vi "animated ranked results.vi"(0 "cases CSV":string[][](array[string]), 5 "US data":T1, 7 "Populations":i32[](array[numeric]), 9 "deaths CSV":string[][](array[string]), 11 "Countries":string[](array[string])) -> ()   [LabVIEW 2019]
panel:
  in  "Select Country":u16(ring) items=["Afghanistan", "Albania", "Algeria", "Andorra", "Angola", "Antigua and Barbuda", "Argentina", "Armenia", "Australia, Australian Capital Territory", "Australia, New South Wales", "Australia, Northern Territory", "Australia, Queensland", "Australia, South Australia", "Australia, Tasmania", "Australia, Victoria", "Australia, Western Australia", "Austria", "Azerbaijan", "Bahamas", "Bahrain", "Bangladesh", "Barbados", "Belarus", "Belgium", "Benin", "Bhutan", "Bolivia", "Bosnia and Herzegovina", "Brazil", "Brunei", "Bulgaria", "Burkina Faso", "Cabo Verde", "Cambodia", "Cameroon", "Canada, Alberta", "Canada, British Columbia", "Canada, Grand Princess", "Canada, Manitoba", "Canada, New Brunswick", "Canada, Newfoundland and Labrador", "Canada, Nova Scotia", "Canada, Ontario", "Canada, Prince Edward Island", "Canada, Quebec", "Canada, Saskatchewan", "Central African Republic", "Chad", "Chile", "China, Anhui", "China, Beijing", "China, Chongqing", "China, Fujian", "China, Gansu", "China, Guangdong", "China, Guangxi", "China, Guizhou", "China, Hainan", "China, Hebei", "China, Heilongjiang", "China, Henan", "China, Hong Kong", "China, Hubei", "China, Hunan", "China, Inner Mongolia", "China, Jiangsu", "China, Jiangxi", "China, Jilin", "China, Liaoning", "China, Macau", "China, Ningxia", "China, Qinghai", "China, Shaanxi", "China, Shandong", "China, Shanghai", "China, Shanxi", "China, Sichuan", "China, Tianjin", "China, Tibet", "China, Xinjiang", "China, Yunnan", "China, Zhejiang", "Colombia", "Congo (Brazzaville)", "Congo (Kinshasa)", "Costa Rica", "Cote d'Ivoire", "Croatia", "Diamond Princess", "Cuba", "Cyprus", "Czechia", "Denmark, Faroe Islands", "Denmark, Greenland", "Denmark", "Djibouti", "Dominican Republic", "Ecuador", "Egypt", "El Salvador", "Equatorial Guinea", "Eritrea", "Estonia", "Eswatini", "Ethiopia", "Fiji", "Finland", "France, French Guiana", "France, French Polynesia", "France, Guadeloupe", "France, Mayotte", "France, New Caledonia", "France, Reunion", "France, Saint Barthelemy", "France, St Martin", "France, Martinique", "France", "Gabon", "Gambia", "Georgia", "Germany", "Ghana", "Greece", "Guatemala", "Guinea", "Guyana", "Haiti", "Holy See", "Honduras", "Hungary", "Iceland", "India", "Indonesia", "Iran", "Iraq", "Ireland", "Israel", "Italy", "Jamaica", "Japan", "Jordan", "Kazakhstan", "Kenya", "\"Korea", "Kuwait", "Kyrgyzstan", "Latvia", "Lebanon", "Liberia", "Liechtenstein", "Lithuania", "Luxembourg", "Madagascar", "Malaysia", "Maldives", "Malta", "Mauritania", "Mauritius", "Mexico", "Moldova", "Monaco", "Mongolia", "Montenegro", "Morocco", "Namibia", "Nepal", "Netherlands, Aruba", "Netherlands, Curacao", "Netherlands, Sint Maarten", "Netherlands", "New Zealand", "Nicaragua", "Niger", "Nigeria", "North Macedonia", "Norway", "Oman", "Pakistan", "Panama", "Papua New Guinea", "Paraguay", "Peru", "Philippines", "Poland", "Portugal", "Qatar", "Romania", "Russia", "Rwanda", "Saint Lucia", "Saint Vincent and the Grenadines", "San Marino", "Saudi Arabia", "Senegal", "Serbia", "Seychelles", "Singapore", "Slovakia", "Slovenia", "Somalia", "South Africa", "Spain", "Sri Lanka", "Sudan", "Suriname", "Sweden", "Switzerland", "Taiwan*", "Tanzania", "Thailand", "Togo", "Trinidad and Tobago", "Tunisia", "Turkey", "Uganda", "Ukraine", "United Arab Emirates", "United Kingdom, Bermuda", "United Kingdom, Cayman Islands", "United Kingdom, Channel Islands", "United Kingdom, Gibraltar", "United Kingdom, Isle of Man", "United Kingdom, Montserrat", "United Kingdom", "Uruguay", "US", "Uzbekistan", "Venezuela", "Vietnam", "Zambia", "Zimbabwe", "Canada, Diamond Princess", "Dominica", "Grenada", "Mozambique", "Syria", "Timor-Leste", "Belize", "Canada, Recovered", "Laos", "Libya", "West Bank and Gaza", "Guinea-Bissau", "Mali", "Saint Kitts and Nevis", "Canada, Northwest Territories", "Canada, Yukon", "Kosovo", "Burma", "United Kingdom, Anguilla", "United Kingdom, British Virgin Islands", "United Kingdom, Turks and Caicos Islands", "MS Zaandam", "Botswana", "Burundi", "Sierra Leone", " Sint Eustatius and Saba\", \"Bonaire", "Malawi", "United Kingdom, Falkland Islands (Malvinas)", "France, Saint Pierre and Miquelon", "South Sudan", "Western Sahara", "Sao Tome and Principe", "Yemen", "Comoros", "Tajikistan", "American Samoa", "Guam", "Northern Mariana Islands", "Puerto Rico", "Virgin Islands", "Alabama", "Alaska", "Arizona", "Arkansas", "California", "Colorado", "Connecticut", "Delaware", "Florida", "Georgia", "Hawaii", "Idaho", "Illinois", "Indiana", "Iowa", "Kansas", "Kentucky", "Louisiana", "Maine", "Maryland", "Massachusetts", "Michigan", "Minnesota", "Mississippi", "Missouri", "Montana", "Nebraska", "Nevada", "New Hampshire", "New Jersey", "New Mexico", "New York", "North Carolina", "North Dakota", "Ohio", "Oklahoma", "Oregon", "Pennsylvania", "Rhode Island", "South Carolina", "South Dakota", "Tennessee", "Texas", "Utah", "Vermont", "Virginia", "Washington", "West Virginia", "Wisconsin", "Wyoming"]
  out "XY Graph":cluster{i32[], i32[]}[](graph)
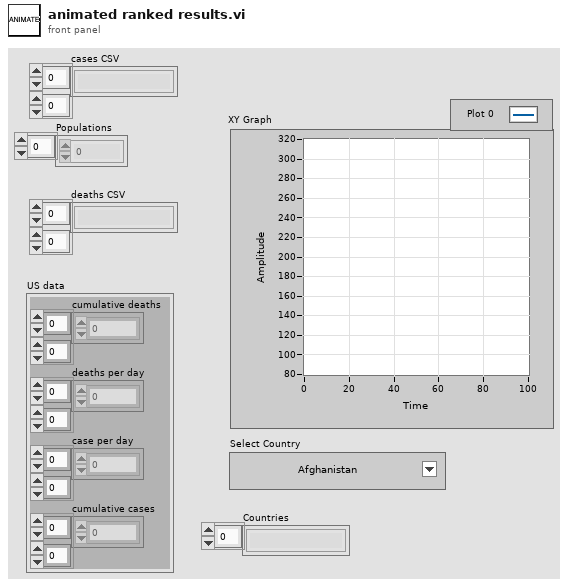
[diagram p1: front panel]
types:
  T1 = cluster{"cumulative deaths":i32[][], "deaths per day":i32[][], "case per day":i32[][], "cumulative cases":i32[][]}
  T2 = cluster{"new deaths per 1M yesterday":dbl, "country index":i32}
  T3 = cluster{"new cases per 1M yesterday":dbl, "country index":i32}
  T4 = cluster{"new deaths yesterday":i32, "country index":i32}
  T5 = cluster{"cumalative cases":i32, "country index":i32}
  T6 = cluster{"cumalative cases":i32, "country index":i32}[]
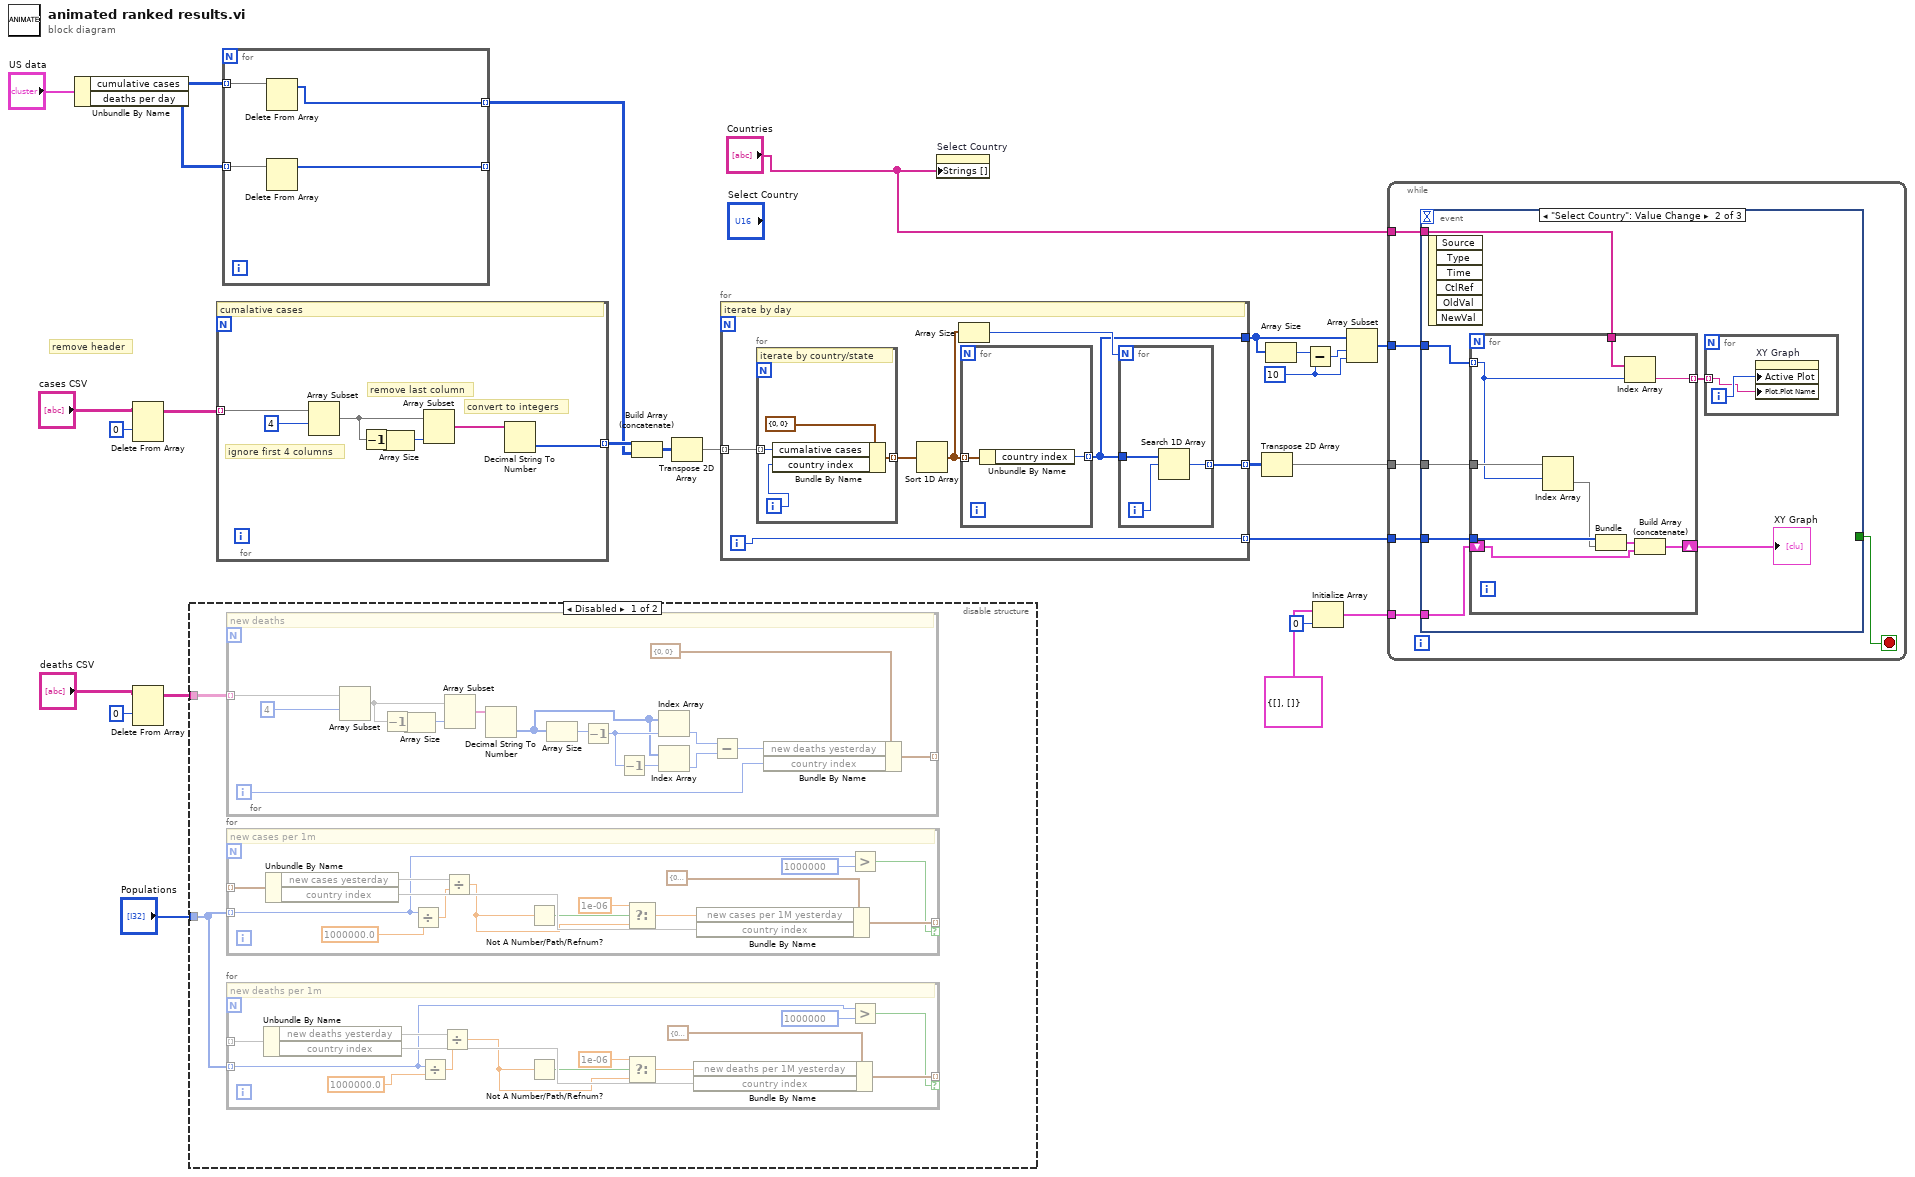
[diagram p0: block diagram]
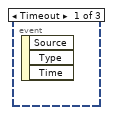
[diagram p2: hidden frame]
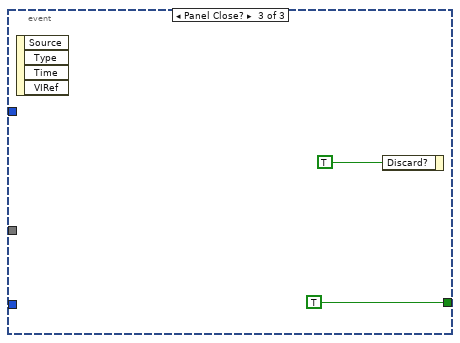
[diagram p3: hidden frame]
diagram:
  w6 = 10 ("y")
  # "remove header"
  n1 = Unbundle By Name("US data") -> ("cumulative cases"=w18:i32[][], "deaths per day"=w17:i32[][])
  n2 = Delete From Array(array="cases CSV", index (row)=0) -> (array with subset deleted=w25:string[][])  [unwired: 2 in, 1 out]
  n3 = Delete From Array(array="deaths CSV", index (row)=0) -> (array with subset deleted=w21:string[][])  [unwired: 2 in, 1 out]
  n4 = disable-structure shown="Disabled" {
    disable-tunnel: w21 -> [w31 _]
    disable-tunnel: "Populations" -> [w30 _]
    frame Disabled {
      n5 = for {
        tunnel: w31 -> [w64] mode=indexing
        tunnel: [w61] -> w29 mode=indexing
        i -> [w60]
        # "new deaths"
        n6 = Array Subset(array=w64, index=4) -> (w72:string[])  [unwired: 1 in]
        n7 = Array Size(array=w72) -> (size(s)=w73:i32)
        n8 = Decrement(x=w73) -> (x-1=w71:i32)
        n9 = Array Subset(array=w72, length=w71) -> (w74:string[])  [unwired: 1 in]
        n10 = Decimal String To Number(string=w74) -> (number=w65:i32[])  [unwired: 2 in, 1 out]
        n11 = Array Size(array=w65) -> (size(s)=w66:i32)
        n12 = Decrement(x=w66) -> (x-1=w69:i32)
        n13 = Decrement(x=w69) -> (x-1=w70:i32)
        n14 = Index Array(array=w65, index=w69) -> (element=w67:i32)
        n15 = Index Array(array=w65, index=w70) -> (element=w68:i32)
        n16 = Subtract(x=w67, y=w68) -> (x-y=w63:i32)
        n17 = Bundle By Name(cluster=T4 {"new deaths yesterday"=0, "country index"=0}, "new deaths yesterday"=w63, "country index"=w60) -> (w61:T4)
      }
      n18 = for {
        tunnel: [w59] -> w28 mode=indexing
        tunnel: w30 -> [w48] mode=indexing
        tunnel: [w56] -> _ mode=indexing if=w46
        # "new cases per 1m"
        n19 = Unbundle By Name(w59) -> ("new cases yesterday"=w54, "country index"=w57)
        n20 = Divide(x=w48, y=1000000.0) -> (x/y=w53:dbl)
        n21 = Divide(x=w54, y=w53) -> (x/y=w50:dbl)
        n22 = Not A Number/Path/Refnum?(number/path/refnum=w50) -> (NaN/Path/Refnum?=w51:bool)
        n23 = Select(t=1e-06, s=w51, f=w50) -> (s? t:f=w49:dbl)
        n24 = Bundle By Name(cluster=T3 {"new cases per 1M yesterday"=0.0, "country index"=0}, "new cases per 1M yesterday"=w49, "country index"=w57) -> (w56:T3)
        n25 = Greater?(x=w48, y=1000000) -> (0:w46:bool)
      }
      n26 = for {
        tunnel: [w45] -> w27 mode=indexing
        tunnel: w30 -> [w32] mode=indexing
        tunnel: [w44] -> _ mode=indexing if=w33
        # "new deaths per 1m"
        n27 = Unbundle By Name(w45) -> ("new deaths yesterday"=w41, "country index"=w42)
        n28 = Divide(x=w32, y=1000000.0) -> (x/y=w39:dbl)
        n29 = Divide(x=w41, y=w39) -> (x/y=w37:dbl)
        n30 = Not A Number/Path/Refnum?(number/path/refnum=w37) -> (NaN/Path/Refnum?=w38:bool)
        n31 = Select(t=1e-06, s=w38, f=w37) -> (s? t:f=w36:dbl)
        n32 = Bundle By Name(cluster=T2 {"new deaths per 1M yesterday"=0.0, "country index"=0}, "new deaths per 1M yesterday"=w36, "country index"=w42) -> (w44:T2)
        n33 = Greater?(x=w32, y=1000000) -> (0:w33:bool)
      }
    }
    frame Enabled {
    }
  }
  n34 = for {
    tunnel: w25 -> [w77] mode=indexing
    tunnel: [w76] -> w16 mode=indexing
    # "remove last column"
    # "convert to integers"
    # "ignore first 4 columns"
    # "cumalative cases"
    n35 = Array Subset(array=w77, index=4) -> (w80:string[])  [unwired: 1 in]
    n36 = Array Size(array=w80) -> (size(s)=w78:i32)
    n37 = Decrement(x=w78) -> (x-1=w79:i32)
    n38 = Array Subset(array=w80, length=w79) -> (w81:string[])  [unwired: 1 in]
    n39 = Decimal String To Number(string=w81) -> (number=w76:i32[])  [unwired: 2 in, 1 out]
  }
  n40 = for {
    tunnel: w18 -> [w86] mode=indexing
    tunnel: w17 -> [w85] mode=indexing
    tunnel: [w84] -> w15 mode=indexing
    tunnel: [w83] -> _ mode=indexing
    n41 = Delete From Array(array=w86) -> (array with subset deleted=w84:i32[])  [unwired: 2 in, 1 out]
    n42 = Delete From Array(array=w85) -> (array with subset deleted=w83:i32[])  [unwired: 2 in, 1 out]
  }
  n43 = Build Array (concatenate)(w16, w15) -> (w14:i32[][])
  n44 = Transpose 2D Array(2D array=w14) -> (transposed array=w13:i32[][])
  n45 = for {
    tunnel: w13 -> [w93] mode=indexing
    tunnel: [w89] -> w12 mode=indexing
    tunnel: [w88] -> w10 mode=indexing
    tunnel: [w87] -> w9
    i -> [w88]
    # "iterate by day"
    n46 = for {
      tunnel: w93 -> [w102] mode=indexing
      tunnel: [w99] -> w92 mode=indexing
      i -> [w100]
      # "iterate by country/state"
      n47 = Bundle By Name(cluster=T5 {"cumalative cases"=0, "country index"=0}, "cumalative cases"=w102, "country index"=w100) -> (w99:T5)
    }
    n48 = Sort 1D Array(array=w92) -> (sorted array=w91:T6)
    n49 = Array Size(array=w91) -> (size(s)=w90:i32)
    n50 = for {
      tunnel: w91 -> [w98] mode=indexing
      tunnel: [w97] -> w87 mode=indexing
      n51 = Unbundle By Name(w98) -> ("country index"=w97:i32)
    }
    n52 = for {
      N: w90 -> [_]
      tunnel: w87 -> [w96]
      tunnel: [w94] -> w89 mode=indexing
      i -> [w95]
      n53 = Search 1D Array(1D array=w96, element=w95) -> (index of element=w94:i32)  [unwired: 1 in]
    }
  }
  n54 = property on="Select Country" class="Ring (strict)"("Strings []"="Countries") -> ()  [unwired: 2 in, 2 out]
  n55 = Transpose 2D Array(2D array=w12) -> (transposed array=w11:i32[][])
  n56 = Array Size(array=w9) -> (size(s)=w8:i32)
  n57 = Subtract(x=w8, y=w6) -> (x-y=w7:i32)
  n58 = Initialize Array(cluster{i32[], i32[]} {[], []}, 0 ("dimension size")) -> (w2:cluster{i32[], i32[]}[])
  n59 = Array Subset(array=w9, index=w7, length=w6) -> (w5:i32[])
  n60 = while {
    tunnel: w11 -> [w108]
    tunnel: w10 -> [w107]
    tunnel: w5 -> [w105]
    tunnel: w2 -> [w104]
    tunnel: "Countries" -> [w103]
    stop <- w106 stop-if-true
    n61 = event shown="[1] \"Select Country\": Value Change" {
      selector: _ -> [_ _ _]
      dyn-events: _ -> [_ _ _]
      timeout: _ -> [_ _ _]
      tunnel: w108 -> [_ w115 _]
      tunnel: w107 -> [_ w114 _]
      tunnel: [_ _ TRUE] -> w106
      tunnel: w105 -> [_ w113 _]
      tunnel: w104 -> [_ w111 _]
      tunnel: w103 -> [_ w110 _]
      event Timeout {
        n62 = event-data() -> ()  [unwired: 1 in, 3 out]
      }
      event "Select Country": Value Change {
        n63 = event-data() -> ()  [unwired: 1 in, 6 out]
        n64 = for {
          tunnel: w115 -> [w126]
          tunnel: w114 -> [w125]
          tunnel: w113 -> [w119] mode=indexing
          shift-right: [w122] -> w112
          shift-left: w111 -> [w121]
          tunnel: w110 -> [w120]
          tunnel: [w118] -> w109 mode=indexing
          n65 = Index Array(array=w126, index (row)=w119) -> (element=w124:i32[])  [unwired: 1 in]
          n66 = Bundle(w125, w124) -> (w123:cluster{i32[], i32[]})  [unwired: 1 in]
          n67 = Index Array(array=w120, index=w119) -> (element=w118:string)
          n68 = Build Array (concatenate)(w123, w121) -> (w122:cluster{i32[], i32[]}[])
        }
        "XY Graph" <- w112
        n69 = for {
          tunnel: w109 -> [w116] mode=indexing
          i -> [w117]
          n70 = property on="XY Graph" class="XYGraph (strict)"("Active Plot"=w117, "Plot.Plot Name"=w116) -> ()  [unwired: 2 in, 2 out]
        }
      }
      event Panel Close? {
        n71 = event-data() -> ()  [unwired: 1 in, 4 out]
        n72 = event-data("Discard?"=TRUE) -> ()  [unwired: 1 in, 1 out]
      }
    }
  }
